vi "InitaliseODrive.vi"(8 "error in (no error)":errorcluster, 11 "FPGA Interface in":refnum<k20>) -> (0 "error out":errorcluster, 1 "Encoder Index Position":i16, 3 "FPGA Interface out":refnum<k20>)   [LabVIEW 2016]
uses:
  <vilib>/Utility/error.llb/Error Cluster From Error Code.vi
  <vilib>/rvi/errors/niLvFpgaAdjustHostInterfaceError.vi
  <vilib>/RVI Host/nirviSupport.llb/nirviErrorClusterFromErrorCode.vi
  <vilib>/rvi/interface/nirviMethod/nirviMethod.xnode
  <vilib>/rvi/interface/nirviReadWriteControl/nirviReadWriteControl.xnode
  NiFpgaLv.dll
  <vilib>/rvi/interface/Simulation/niFpgaSimulationCallBeginRW.vi
  <vilib>/rvi/errors/niLvFpgaMergeErrorWithErrorCode.vi
  <vilib>/FPGAPlugInAG/Dynamic/niLvFpga_WriteFifo_Dynamic.vi
  <vilib>/rvi/interface/nirviMethod/StockFPGA_InlinedMethodWaitForSingleIRQ.vi
  <vilib>/FPGAPlugInAG/Dynamic/niLvFpga_WaitOnIrq_Dynamic.vi
  <vilib>/FPGAPlugInAG/Dynamic/niLvFpga_AcknowledgeIrq_Dynamic.vi
  <vilib>/FPGAPlugInAG/Dynamic/niLvFpga_StartFifo_Dynamic.vi
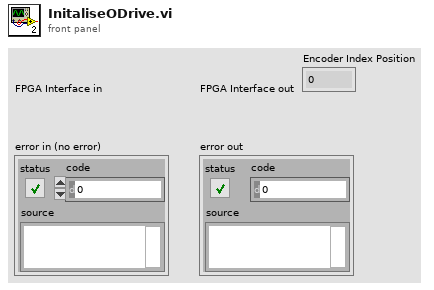
[diagram p1: front panel]
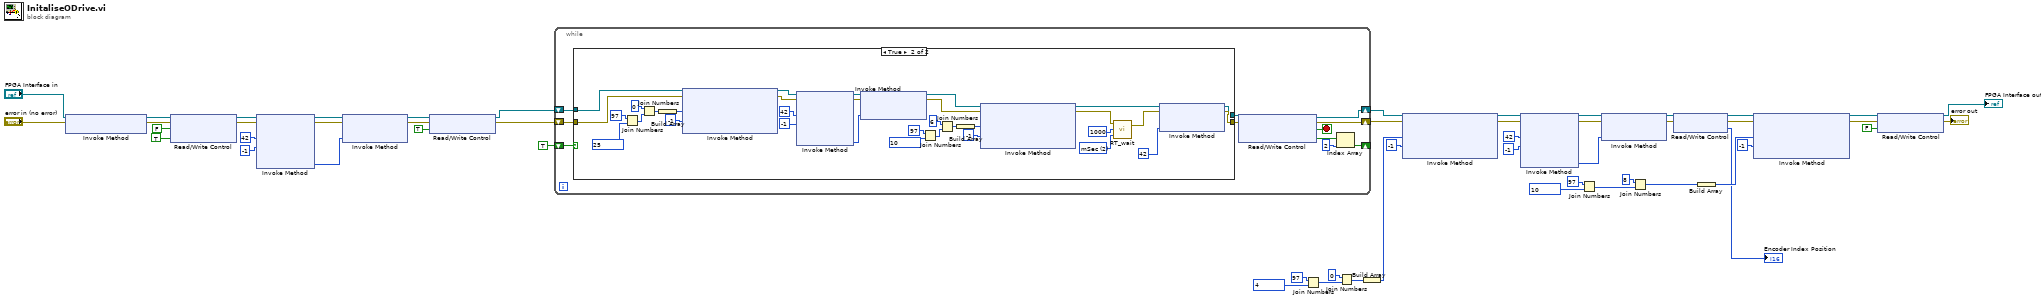
[diagram p0: block diagram]
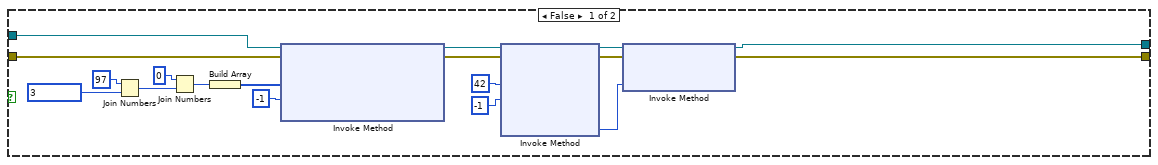
[diagram p2: hidden frame]
diagram:
  n1 = xnode "Invoke Method"("FPGA VI Reference In"="FPGA Interface in", "error in"="error in (no error)") -> ("FPGA VI Reference Out"=w46:refnum<k20>, "error out"=w47:errorcluster)
  n2 = xnode "Read/Write Control"("FPGA VI Reference In"=w46, "error in"=w47, "ODrive RT Control"=FALSE, "MotorsON"=TRUE) -> ("FPGA VI Reference Out"=w20:refnum<k20>, "error out"=w19:errorcluster)
  n3 = xnode "Invoke Method"("FPGA VI Reference In"=w20, "error in"=w19, "IRQ Number(s)"=42, "Timeout (ms)"=-1) -> ("FPGA VI Reference Out"=w25:refnum<k20>, "error out"=w22:errorcluster, "IRQ(s) Asserted"=w23:i32)  [unwired: 1 out]
  n4 = xnode "Invoke Method"("FPGA VI Reference In"=w25, "error in"=w22, "IRQ Number(s)"=w23) -> ("FPGA VI Reference Out"=w17:refnum<k20>, "error out"=w18:errorcluster)
  n5 = xnode "Read/Write Control"("FPGA VI Reference In"=w17, "error in"=w18, "ODrive RT Control"=TRUE) -> ("FPGA VI Reference Out"=w1:refnum<k20>, "error out"=w2:errorcluster)
  n6 = while {
    shift-right: [w63] -> w37
    shift-left: w2 -> [w60]
    shift-right: [w62] -> w36
    shift-left: w1 -> [w59]
    shift-right: [w58] -> _
    shift-left: TRUE -> [w55]
    stop <- w61 stop-if-true
    n7 = case shown="True" w55 {
      tunnel: w60 -> [w74 w95]
      tunnel: w59 -> [w73 w94]
      tunnel: [w65 w89] -> w53
      tunnel: [w64 w88] -> w54
      frame False {
        n8 = Join Numbers(hi=u8 97, lo=u8 3) -> ((hi.lo)=w79:u16)
        n9 = Join Numbers(hi=u16 0, lo=w79) -> ((hi.lo)=w77:u32)
        n10 = Build Array(w77) -> (w76:u32[])
        n11 = xnode "Invoke Method"("FPGA VI Reference In"=w73, "error in"=w74, "Data"=w76, "Timeout (ms)"=-1) -> ("FPGA VI Reference Out"=w66:refnum<k20>, "error out"=w67:errorcluster)  [unwired: 1 out]
        n12 = xnode "Invoke Method"("FPGA VI Reference In"=w66, "error in"=w67, "IRQ Number(s)"=42, "Timeout (ms)"=-1) -> ("FPGA VI Reference Out"=w69:refnum<k20>, "error out"=w71:errorcluster, "IRQ(s) Asserted"=w70:i32)  [unwired: 1 out]
        n13 = xnode "Invoke Method"("FPGA VI Reference In"=w69, "error in"=w71, "IRQ Number(s)"=w70) -> ("FPGA VI Reference Out"=w64:refnum<k20>, "error out"=w65:errorcluster)
      }
      frame True {
        w86 = u16 2 items=["Ticks", "uSec", "mSec"] ("Counter Units")
        n14 = Join Numbers(hi=u8 97, lo=u8 25) -> ((hi.lo)=w105:u16)
        n15 = Join Numbers(hi=u16 0, lo=w105) -> ((hi.lo)=w103:u32)
        n16 = Build Array(w103) -> (w102:u32[])
        n17 = xnode "Invoke Method"("FPGA VI Reference In"=w94, "error in"=w95, "Data"=w102, "Timeout (ms)"=-1) -> ("FPGA VI Reference Out"=w92:refnum<k20>, "error out"=w93:errorcluster)  [unwired: 1 out]
        n18 = xnode "Invoke Method"("FPGA VI Reference In"=w92, "error in"=w93, "IRQ Number(s)"=42, "Timeout (ms)"=-1) -> ("FPGA VI Reference Out"=w99:refnum<k20>, "error out"=w97:errorcluster, "IRQ(s) Asserted"=w98:i32)  [unwired: 1 out]
        n19 = xnode "Invoke Method"("FPGA VI Reference In"=w99, "error in"=w97, "IRQ Number(s)"=w98) -> ("FPGA VI Reference Out"=w90:refnum<k20>, "error out"=w91:errorcluster)
        n20 = Join Numbers(hi=u8 97, lo=u8 10) -> ((hi.lo)=w112:u16)
        n21 = Join Numbers(hi=u16 6, lo=w112) -> ((hi.lo)=w110:u32)
        n22 = Build Array(w110) -> (w109:u32[])
        n23 = xnode "Invoke Method"("FPGA VI Reference In"=w90, "error in"=w91, "Data"=w109, "Timeout (ms)"=-1) -> ("FPGA VI Reference Out"=w82:refnum<k20>, "error out"=w84:errorcluster)  [unwired: 1 out]
        n24 = call "RT_wait.vi"("Counter Units"=w86, "Count(mSec)"=u32 1000, "error in (no error)"=w84) -> ("error out"=w83:errorcluster)  [unwired: 1 in, 1 out]
        n25 = xnode "Invoke Method"("FPGA VI Reference In"=w82, "error in"=w83, "IRQ Number(s)"=42) -> ("FPGA VI Reference Out"=w88:refnum<k20>, "error out"=w89:errorcluster)
      }
    }
    n26 = xnode "Read/Write Control"("FPGA VI Reference In"=w54, "error in"=w53) -> ("FPGA VI Reference Out"=w62:refnum<k20>, "error out"=w63:errorcluster, "ODrive Encoder ready"=w61:bool, "ODrive Error Flags"=w57:bool[])
    n27 = Index Array(array=w57, index=2) -> (element=w58:bool)
  }
  n28 = Join Numbers(hi=u8 97, lo=u8 4) -> ((hi.lo)=w41:u16)
  n29 = Join Numbers(hi=u16 0, lo=w41) -> ((hi.lo)=w39:u32)
  n30 = Build Array(w39) -> (w38:u32[])
  n31 = xnode "Invoke Method"("FPGA VI Reference In"=w36, "error in"=w37, "Data"=w38, "Timeout (ms)"=-1) -> ("FPGA VI Reference Out"=w29:refnum<k20>, "error out"=w30:errorcluster)  [unwired: 1 out]
  n32 = xnode "Invoke Method"("FPGA VI Reference In"=w29, "error in"=w30, "IRQ Number(s)"=42, "Timeout (ms)"=-1) -> ("FPGA VI Reference Out"=w34:refnum<k20>, "error out"=w31:errorcluster, "IRQ(s) Asserted"=w32:i32)  [unwired: 1 out]
  n33 = Join Numbers(hi=u8 97, lo=u8 10) -> ((hi.lo)=w13:u16)
  n34 = xnode "Invoke Method"("FPGA VI Reference In"=w34, "error in"=w31, "IRQ Number(s)"=w32) -> ("FPGA VI Reference Out"=w27:refnum<k20>, "error out"=w28:errorcluster)
  n35 = Join Numbers(hi=u16 8, lo=w13) -> ((hi.lo)=w15:u32)
  n36 = xnode "Read/Write Control"("FPGA VI Reference In"=w27, "error in"=w28) -> ("FPGA VI Reference Out"=w10:refnum<k20>, "error out"=w9:errorcluster, "Position Axis1"=→"Encoder Index Position":i16)
  n37 = Build Array(w15) -> (w16:u32[])
  n38 = xnode "Invoke Method"("FPGA VI Reference In"=w10, "error in"=w9, "Data"=w16, "Timeout (ms)"=-1) -> ("FPGA VI Reference Out"=w8:refnum<k20>, "error out"=w7:errorcluster)  [unwired: 1 out]
  n39 = xnode "Read/Write Control"("FPGA VI Reference In"=w8, "error in"=w7, "ODrive RT Control"=FALSE) -> ("FPGA VI Reference Out"=→"FPGA Interface out":refnum<k20>, "error out"=→"error out":errorcluster)
